vi "NI Rapid Read.vi"(4 "lines per plane":u16, 5 "Reverse?":bool, 6 "error in":errorcluster, 7 "rf points per line":u16, 8 "Motion Board ID":T1=1 min=1 max=32 step=1, 9 "Inst ID":refnum<k15>) -> (0 "error out":errorcluster, 1 "Dig Word Size":u16, 3 "Array":i16[][](array[numeric]))   [LabVIEW 2022 SP3]
uses:
  <vilib>/Motion/FlexMotion/CustomControls/CustomControls.llb/Mask (8 axes).flx
  <vilib>/Motion/FlexMotion/FunctionsVIs/MotionIO.llb/Set Inhibit MOMO (8 axes).flx
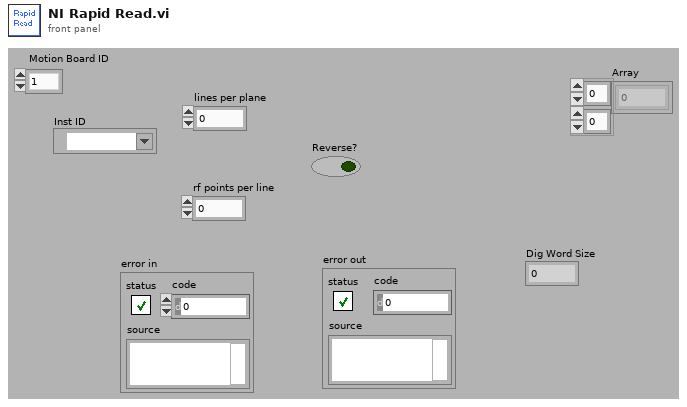
[diagram p1: front panel]
types:
  T1 = typedef "Board Id" = u8
  T2 = typedef "Mask (8 axes).flx" = cluster{"1":bool, "2":bool, "3":bool, "4":bool, "5":bool, "6":bool, "7":bool, "8":bool}
  T3 = typedef "Bd Id Out" = u8
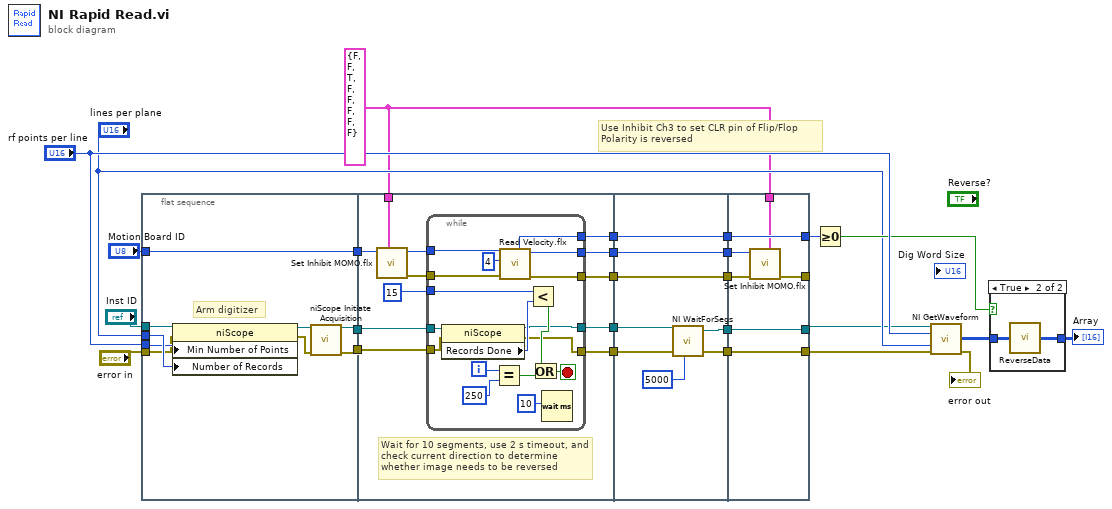
[diagram p0: block diagram]
diagram:
  w6 = T2 {"1"=FALSE, "2"=FALSE, "3"=TRUE, "4"=FALSE, "5"=FALSE, "6"=FALSE, "7"=FALSE, "8"=FALSE} ("Must On (False)")
  # "Use Inhibit Ch3 to set CLR pin of Flip/Flop\nPolarity is reversed"
  n1 = flat-sequence {
    tunnel: "Motion Board ID" -> [w35]
    tunnel: [w33] -> w5
    tunnel: "Inst ID" -> [w28]
    tunnel: [w34] -> w4
    tunnel: "error in" -> [w27]
    tunnel: "lines per plane" -> [w30]
    tunnel: "rf points per line" -> [w29]
    tunnel: [w35] -> w3
    tunnel: [w46] -> w13
    tunnel: [w47] -> w12
    tunnel: [w44] -> w11
    tunnel: [w43] -> w9
    tunnel: [w42] -> w10
    tunnel: w5 -> [w41]
    tunnel: w4 -> [w40]
    tunnel: w6 -> [w37]
    tunnel: w3 -> [w36]
    tunnel: w13 -> [w71]
    tunnel: w12 -> [w66]
    tunnel: w9 -> [w70]
    tunnel: [w73] -> w23
    tunnel: [w72] -> w22
    tunnel: [w70] -> w21
    tunnel: [w69] -> w20
    tunnel: w11 -> [w69]
    tunnel: [w68] -> w19
    tunnel: w10 -> [w68]
    tunnel: w23 -> [w80]
    tunnel: w22 -> [w79]
    tunnel: w21 -> [w78]
    tunnel: w20 -> [w77]
    tunnel: w19 -> [w76]
    tunnel: w6 -> [w74]
    tunnel: [w80] -> w1
    tunnel: [w79] -> w2
    tunnel: [w78] -> w25
    tunnel: [w75] -> _
    frame #0 {
      # "Arm digitizer"
      n2 = property class="niScope"(reference=w28, error in=w27, "Min Number of Points"=w29, "Number of Records"=w30) -> (reference out=w32:refnum<k15>, error out=w31:errorcluster)
      n3 = call <instrlib>:"niScope Initiate Acquisition.vi"("instrument handle"=w32, "error in"=w31) -> ("instrument handle out"=w33:refnum<k15>, "error out"=w34:errorcluster)  [unwired: 12 out]
    }
    frame #1 {
      # "Wait for 10 segments, use 2 s timeout, and check current direction to determine whether image needs to be reversed"
      n4 = call-poly <vilib>:"Set Inhibit MOMO.flx"("Must On (False)"=w37, "Board ID"=w36) -> ("error out"=w39:errorcluster, "Bd ID Out"=w38:T3)  [unwired: 2 in, 4 out]
      n5 = while {
        tunnel: [w48] -> w46
        tunnel: w40 -> [w51]
        tunnel: w41 -> [w52]
        tunnel: [w49] -> w47
        tunnel: 15 -> [w65]
        tunnel: w38 -> [w57]
        tunnel: w39 -> [w56]
        tunnel: [w55] -> w44
        tunnel: [w54] -> w43
        tunnel: [w53] -> w42
        i -> [w64]
        stop <- w60 stop-if-true
        n6 = property class="niScope"(reference=w52, error in=w51) -> (reference out=w49:refnum<k15>, error out=w48:errorcluster, "Records Done"=w50:i32)
        n7 = Equal?(x=w64, y=250) -> (x = y?=w62:bool)
        n8 = call <vilib>:"Read Velocity.flx"("error in (no error)"=w56, "Axis or Vector Space"=4, "Board ID"=w57) -> ("error out"=w53:errorcluster, "Bd ID Out"=w55:T3, "Filtered Velocity"=w54:i32)  [unwired: 4 out]
        n9 = Less?(x=w65, y=w50) -> (x < y?=w61:bool)
        n10 = Or(x=w61, y=w62) -> (x .or. y?=w60:bool)
        n11 = Wait (ms)(milliseconds to wait=10) -> ()  [unwired: 1 out]
      }
    }
    frame #2 {
      n12 = call "NI WaitForSegs.vi"("NI ID"=w66, "error in"=w71, "Timeout"=5000) -> ("Instrument ID"=w72:refnum<k15>, "error out"=w73:errorcluster)  [unwired: 1 in, 2 out]
    }
    frame #3 {
      n13 = call-poly <vilib>:"Set Inhibit MOMO.flx"("Must Off (False)"=w74, "error in (no error)"=w76, "Board ID"=w77) -> ("error out"=w75:errorcluster)  [unwired: 1 in, 5 out]
    }
  }
  n14 = Greater Or Equal To 0?(x=w25) -> (x >= 0?=w15:bool)
  n15 = call "NI GetWaveform.vi"("Acq ID In"=w2, "Num Samps"="rf points per line", "Num Segs"="lines per plane", "error in"=w1) -> ("Acquired Waveform16 bit"=w8:i8[][], "error out"=→"error out":errorcluster)  [unwired: 6 in, 4 out]
  n16 = case shown="True" w15 {
    tunnel: w8 -> [w81 w83]
    tunnel: [w81 w82] -> w7
    frame False {
    }
    frame True {
      n17 = call "ReverseData.vi"("Array in"=w83) -> ("Array out"=w82:i16[][])
    }
  }
  "Array" <- w7
